vi "Write enable module timing info.vi"(8 "error in":errorcluster, 10 "enable module timing info":bool, 11 "Standard Engine Configuration in":refnum<class "Standard Engine Configuration.lvclass">) -> (0 "error out":errorcluster, 3 "Standard Engine Configuration out":refnum<class "Standard Engine Configuration.lvclass">)   [LabVIEW 2013, in "Standard Engine Configuration.lvclass"]
uses:
  Standard Engine Configuration.lvclass
  Standard Engine Configuration.lvclass/Standard Engine Configuration.ctl
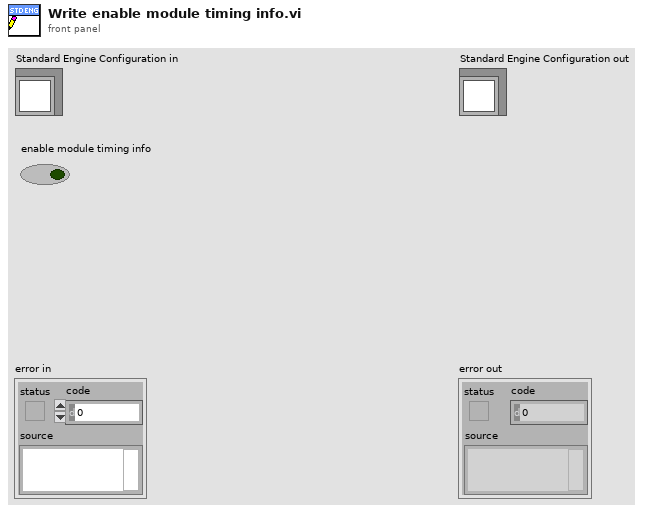
[diagram p1: front panel]
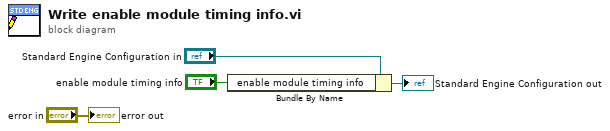
[diagram p0: block diagram]
diagram:
  n1 = Bundle By Name(cluster="Standard Engine Configuration in", "enable module timing info"="enable module timing info") -> (→"Standard Engine Configuration out":refnum<class "Standard Engine Configuration.lvclass">)
  "error out" <- "error in"
